vi "Get Illuminance Callback Threshold.vi"(8 "error in (no error)":errorcluster, 11 "Ambient Light Bricklet in":refnum<class "Ambient Light Bricklet.lvclass">) -> (0 "error out":errorcluster, 1 "max":i16, 2 "min":i16, 3 "Ambient Light Bricklet out":refnum<class "Ambient Light Bricklet.lvclass">, 5 "Callback Option":T1)   [LabVIEW 2011, in "Tinkerforge.lvlib" / "Ambient Light Bricklet.lvclass"]
doc: "This VI returns the threshold configuration of the illuminance callback."
uses:
  Ambient Light Bricklet.lvclass
  Device/Type Definitions/Callback Option.ctl
  Device/Type Definitions/Callback Threshold.ctl
  Device/Device.lvclass
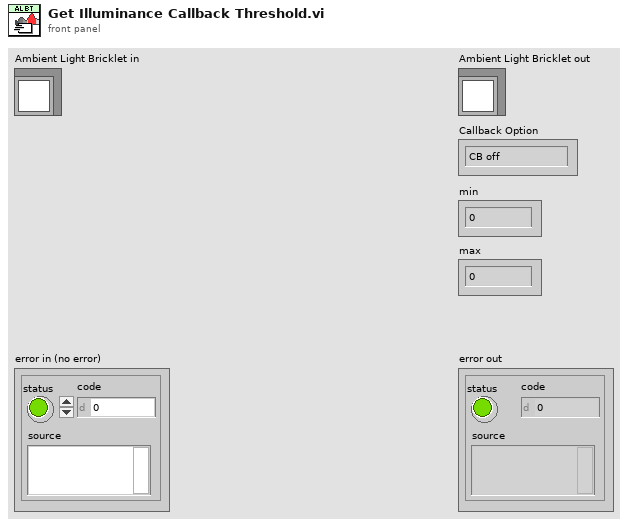
[diagram p1: front panel]
types:
  T1 = typedef "Tinkerforge.lvlib/Device.lvclass/Callback Option.ctl" = enum8{"CB off", "outside range", "inside range", "smaller", "greater"}
  T2 = typedef "Tinkerforge.lvlib/Device.lvclass/Callback Threshold.ctl" = cluster{"Callback Option":T1, "min":i16, "max":i16}
  T3 = typedef "Tinkerforge.lvlib/IP Connection.lvclass/Answer.ctl" = cluster{"Request GUID":string, "Request Type":T4, "Sucessful":bool, "Data":variant, "Error":errorcluster}
  T4 = typedef "Tinkerforge.lvlib/IP Connection.lvclass/Request Type.ctl" = enum8{"Invalid", "Write"}
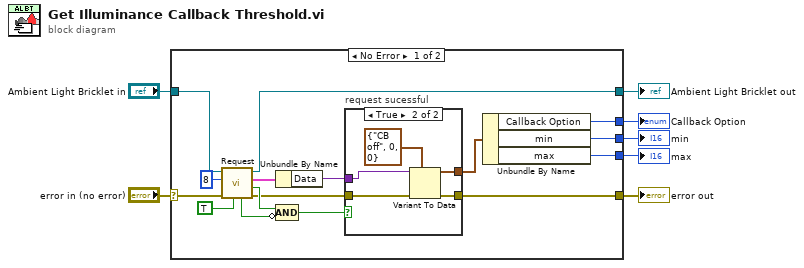
[diagram p0: block diagram]
diagram:
  n1 = case shown="No Error" "error in (no error)" {
    selector: "error in (no error)" -> [w23 w31]
    tunnel: [w12 w31] -> w6
    tunnel: [w21 w30] -> w4
    tunnel: "Ambient Light Bricklet in" -> [w22 w30]
    tunnel: [w10 _] -> w3
    tunnel: [w9 _] -> w2
    tunnel: [w8 _] -> w1
    frame No Error {
      n2 = call "Request.vi"("Response"=TRUE, "error in (no error)"=w23, "Function ID"=u8 8, "Device in"=w22) -> ("error out"=w15:errorcluster, "Sucessful"=w17:bool, "Answer"=w14:T3, "Device out"=w21:refnum<class "Ambient Light Bricklet.lvclass">, "timed out"=w18:bool)  [unwired: 3 in]
      n3 = Unbundle By Name(w14) -> ("Data"=w13:variant)
      n4 = Compound Arithmetic op=AND(w17, invert w18) -> (w16:bool)
      n5 = case "request sucessful" shown="True" w16 {
        tunnel: w15 -> [w24 w29]
        tunnel: w13 -> [_ w28]
        tunnel: [_ w27] -> w11
        tunnel: [w24 w26] -> w12
        frame False {
        }
        frame True {
          n6 = Variant To Data(error in=w29, type=T2 {"Callback Option"=enum."CB off", "min"=0, "max"=0} ("Callback Threshold"), Variant=w28) -> (data=w27:T2, error out=w26:errorcluster)
        }
      }
      n7 = Unbundle By Name(w11) -> ("Callback Option"=w10:T1, "min"=w9:i16, "max"=w8:i16)
    }
    frame Error {
    }
  }
  "error out" <- w6
  "Ambient Light Bricklet out" <- w4
  "Callback Option" <- w3
  "min" <- w2
  "max" <- w1
